vi "Create Event Queue.vi"() -> (0 "Event Queue":refnum<queue>)   [LabVIEW 2022 SP3, in "FlexBlocks Support.lvlib"]
uses:
  FlexBlocks Support.lvlib
  Execution Events.ctl
  Worker Registration.ctl
  Worker Block.ctl
  Block Status with Error.ctl
  Block Status.ctl
  Block State.ctl
  Block Phase.ctl
  Block Command.ctl
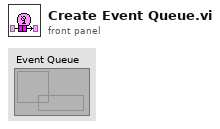
[diagram p1: front panel]
types:
  T1 = typedef "FlexBlocks Support.lvlib/Execution Events.ctl" = cluster{"Registration":refnum<user-event>, "Init":refnum<user-event>, "Run":refnum<user-event>, "Step":refnum<user-event>, "Stop":refnum<user-event>, "Close":refnum<user-event>, "Block Status":refnum<user-event>}
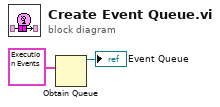
[diagram p0: block diagram]
diagram:
  n1 = Obtain Queue(element data type=T1 {"Registration"=refnum, "Init"=refnum, "Run"=refnum, "Step"=refnum, "Stop"=refnum, "Close"=refnum, "Block Status"=refnum} ("Execution Events")) -> (queue out=→"Event Queue":refnum<queue>)  [unwired: 4 in, 2 out]
